vi "nanocal -- nuclear schottky goodness V5.vi"(5 "action":T1=enum."onlygrads", 6 "parameters IN":map{T2, dbl}(c390), 7 "weighting strategy":T3, 8 "dz/dω IN (V)":cdb[](array[numeric])=[1.7183506006211996e-05+0.0i, 1.7124360968751133e-05+0.0i, 1.7049104347380084e-05+0.0i, 1.700437896335042e-05+0.0i, 1.6984579723285106e-05+0.0i, 1.702277369054923e-05+0.0i, 1.713094025845651e-05+0.0i, 1.734249707866828e-05+0.0i, 1.768320429215342e-05+0.0i, 1.8195281152538477e-05+0.0i, 1.8917228661806973e-05+0.0i, 1.9897834564883332e-05+0.0i, 2.154104046962704e-05+0.0i, 2.3247799321765792e-05+0.0i, 2.5364678450551808e-05+0.0i, 2.8645788781885885e-05+0.0i, 3.204749554800641e-05+0.0i, 3.783559691555022e-05+0.0i, 4.245015867332296e-05+0.0i, 4.909131821431355e-05+0.0i, 5.511821898441184e-05+0.0i, 6.178843506022867e-05+0.0i, 7.1079604965352e-05+0.0i, 7.922304381453334e-05+0.0i, 8.814778883893872e-05+0.0i, 9.806709148886077e-05+0.0i, 0.00011119043245647465+0.0i, 0.00012253184919712196+0.0i, 0.00013777724317049346+0.0i, 0.0001508081004573332+0.0i, 0.00016547294918783876+0.0i, 0.00018003847596605868+0.0i, 0.00019518361086534857+0.0i, 0.00021134179818259658+0.0i, 0.0002372041782935464+0.0i, 0.00025518143132024254+0.0i, 0.0002835129702467886+0.0i, 0.0003060118087631287+0.0i, 0.00032860772064336976+0.0i, 0.0003492674091322389+0.0i, 0.00037498324855458583+0.0i, 0.00040021078021115026+0.0i, 0.00041969942568205823+0.0i, 0.00044367338947118773+0.0i, 0.0004634793607238068+0.0i, 0.00047921028781215815+0.0i, 0.0004880906353641744+0.0i, 0.0004932212623741357+0.0i, 0.000491476456593048+0.0i, 0.000480893803992059+0.0i, 0.0004535995818650303+0.0i, 0.000417087772881063+0.0i, 0.0003564148692854789+0.0i, 0.0003049201646356487+0.0i, 0.00021260191240459413+0.0i, 0.00011714858948470126+0.0i, 1.675457544365132e-05+0.0i, -6.8674075405897e-05+0.0i, -0.000156473047607305+0.0i, -0.00026709373934749337+0.0i, -0.0003544271565676041+0.0i, -0.00047937600197311275+0.0i, -0.0006086290582260493+0.0i, -0.0007031877411848573+0.0i, -0.0007564526901441745+0.0i, -0.000802489180995596+0.0i, -0.0008414596018105983+0.0i, -0.0008809346482248761+0.0i, -0.0009073902840241921+0.0i, -0.0009264953054508651+0.0i, -0.0009405659412141811+0.0i, -0.000951649722530156+0.0i, -0.0009557485581057351+0.0i, -0.0009558464741053665+0.0i, -0.0009509110176922098+0.0i, -0.0009411315169847015+0.0i, -0.0009303400913929496+0.0i, -0.0009171113529290538+0.0i, -0.0009022111527275027+0.0i, -0.0008813746494947608+0.0i, -0.0008581837971946129+0.0i, -0.0008372063466683705+0.0i, -0.0008165626610594428+0.0i, -0.0007901155435838691+0.0i, -0.0007682834352800848+0.0i, -0.000746231015527196+0.0i, -0.0007238798463130141+0.0i, -0.0007015567569177018+0.0i, -0.000679301954671598+0.0i, -0.0006572001413831251+0.0i, -0.000629855254567978+0.0i, -0.0006083942229188815+0.0i, -0.0005768631156754208+0.0i, -0.0005562177438951648+0.0i, -0.0005359092039599222+0.0i, -0.0005145186443378148+0.0i, -0.0004951602053444319+0.0i, -0.00047624970229075174+0.0i, -0.0004577401041527736+0.0i, -0.00043519037796120065+0.0i], 9 "Voltage IN (V)":cdb[](array[numeric])=[1.7183506006211996e-05+0.0i, 1.7124360968751133e-05+0.0i, 1.7049104347380084e-05+0.0i, 1.700437896335042e-05+0.0i, 1.6984579723285106e-05+0.0i, 1.702277369054923e-05+0.0i, 1.713094025845651e-05+0.0i, 1.734249707866828e-05+0.0i, 1.768320429215342e-05+0.0i, 1.8195281152538477e-05+0.0i, 1.8917228661806973e-05+0.0i, 1.9897834564883332e-05+0.0i, 2.154104046962704e-05+0.0i, 2.3247799321765792e-05+0.0i, 2.5364678450551808e-05+0.0i, 2.8645788781885885e-05+0.0i, 3.204749554800641e-05+0.0i, 3.783559691555022e-05+0.0i, 4.245015867332296e-05+0.0i, 4.909131821431355e-05+0.0i, 5.511821898441184e-05+0.0i, 6.178843506022867e-05+0.0i, 7.1079604965352e-05+0.0i, 7.922304381453334e-05+0.0i, 8.814778883893872e-05+0.0i, 9.806709148886077e-05+0.0i, 0.00011119043245647465+0.0i, 0.00012253184919712196+0.0i, 0.00013777724317049346+0.0i, 0.0001508081004573332+0.0i, 0.00016547294918783876+0.0i, 0.00018003847596605868+0.0i, 0.00019518361086534857+0.0i, 0.00021134179818259658+0.0i, 0.0002372041782935464+0.0i, 0.00025518143132024254+0.0i, 0.0002835129702467886+0.0i, 0.0003060118087631287+0.0i, 0.00032860772064336976+0.0i, 0.0003492674091322389+0.0i, 0.00037498324855458583+0.0i, 0.00040021078021115026+0.0i, 0.00041969942568205823+0.0i, 0.00044367338947118773+0.0i, 0.0004634793607238068+0.0i, 0.00047921028781215815+0.0i, 0.0004880906353641744+0.0i, 0.0004932212623741357+0.0i, 0.000491476456593048+0.0i, 0.000480893803992059+0.0i, 0.0004535995818650303+0.0i, 0.000417087772881063+0.0i, 0.0003564148692854789+0.0i, 0.0003049201646356487+0.0i, 0.00021260191240459413+0.0i, 0.00011714858948470126+0.0i, 1.675457544365132e-05+0.0i, -6.8674075405897e-05+0.0i, -0.000156473047607305+0.0i, -0.00026709373934749337+0.0i, -0.0003544271565676041+0.0i, -0.00047937600197311275+0.0i, -0.0006086290582260493+0.0i, -0.0007031877411848573+0.0i, -0.0007564526901441745+0.0i, -0.000802489180995596+0.0i, -0.0008414596018105983+0.0i, -0.0008809346482248761+0.0i, -0.0009073902840241921+0.0i, -0.0009264953054508651+0.0i, -0.0009405659412141811+0.0i, -0.000951649722530156+0.0i, -0.0009557485581057351+0.0i, -0.0009558464741053665+0.0i, -0.0009509110176922098+0.0i, -0.0009411315169847015+0.0i, -0.0009303400913929496+0.0i, -0.0009171113529290538+0.0i, -0.0009022111527275027+0.0i, -0.0008813746494947608+0.0i, -0.0008581837971946129+0.0i, -0.0008372063466683705+0.0i, -0.0008165626610594428+0.0i, -0.0007901155435838691+0.0i, -0.0007682834352800848+0.0i, -0.000746231015527196+0.0i, -0.0007238798463130141+0.0i, -0.0007015567569177018+0.0i, -0.000679301954671598+0.0i, -0.0006572001413831251+0.0i, -0.000629855254567978+0.0i, -0.0006083942229188815+0.0i, -0.0005768631156754208+0.0i, -0.0005562177438951648+0.0i, -0.0005359092039599222+0.0i, -0.0005145186443378148+0.0i, -0.0004951602053444319+0.0i, -0.00047624970229075174+0.0i, -0.0004577401041527736+0.0i, -0.00043519037796120065+0.0i], 10 "ω (rad/sec)":dbl[](array[numeric])=[32012.991918577427, 32390.261658505893, 32466.39798177853, 32499.14340521798, 32517.39286113775, 32529.046092051318, 32537.14525712326, 32543.111142615544, 32547.696343954158, 32551.33675949651, 32554.302325209504, 32556.769142360055, 32558.856995237307, 32560.650202739795, 32562.209843476354, 32563.58125099723, 32564.7987833122, 32565.88895894197, 32566.872575330308, 32567.766175404246, 32568.583086316496, 32569.334166794306, 32570.02835688638, 32570.673085530187, 32571.274580490695, 32571.838104118455, 32572.36813539066, 32572.868514009202, 32573.342552524307, 32573.793126289274, 32574.222746575288, 32574.633618125405, 32575.027687968828, 32575.40668442971, 32575.772149741057, 32576.12546690325, 32576.467883345118, 32576.800529469096, 32577.124435064776, 32577.440543590797, 32577.749724325146, 32578.052781957467, 32578.35046682089, 32578.643482565894, 32578.932492128843, 32579.218126471686, 32579.500987779396, 32579.781656707495, 32580.06069600583, 32580.338656060805, 32580.616078519142, 32580.89350097748, 32581.171461032456, 32581.45050033079, 32581.73116925889, 32582.0140305666, 32582.29966469628, 32582.58867447239, 32582.88169000423, 32583.179375080817, 32583.48243271314, 32583.791613234323, 32584.10772197351, 32584.43162756919, 32584.764273480003, 32585.106690135035, 32585.460007297228, 32585.825472395412, 32586.204468856296, 32586.59853891288, 32587.009410462997, 32587.439030535847, 32587.889604513977, 32588.363642815923, 32588.86402143446, 32589.39405291983, 32589.957576334426, 32590.559071508098, 32591.203800151903, 32591.897990030815, 32592.64907072179, 32593.46598163404, 32594.359581707977, 32595.343197883154, 32596.433373726086, 32597.650906041054, 32599.022313348767, 32600.58195429849, 32602.375161800977, 32604.46301467823, 32606.929831615616, 32609.895397541775, 32613.535812870963, 32618.12101442274, 32624.086899701866, 32632.186064986967, 32643.839295900536, 32662.088751820305, 32694.834175046595, 32770.97049853239]) -> (0 "R norm":dbl=-1.0, 1 "G":dbl=-1.0, 2 "R(ω) out":cdb[](array[numeric])=[1.7183506006211996e-05+0.0i, 1.7124360968751133e-05+0.0i, 1.7049104347380084e-05+0.0i, 1.700437896335042e-05+0.0i, 1.6984579723285106e-05+0.0i, 1.702277369054923e-05+0.0i, 1.713094025845651e-05+0.0i, 1.734249707866828e-05+0.0i, 1.768320429215342e-05+0.0i, 1.8195281152538477e-05+0.0i, 1.8917228661806973e-05+0.0i, 1.9897834564883332e-05+0.0i, 2.154104046962704e-05+0.0i, 2.3247799321765792e-05+0.0i, 2.5364678450551808e-05+0.0i, 2.8645788781885885e-05+0.0i, 3.204749554800641e-05+0.0i, 3.783559691555022e-05+0.0i, 4.245015867332296e-05+0.0i, 4.909131821431355e-05+0.0i, 5.511821898441184e-05+0.0i, 6.178843506022867e-05+0.0i, 7.1079604965352e-05+0.0i, 7.922304381453334e-05+0.0i, 8.814778883893872e-05+0.0i, 9.806709148886077e-05+0.0i, 0.00011119043245647465+0.0i, 0.00012253184919712196+0.0i, 0.00013777724317049346+0.0i, 0.0001508081004573332+0.0i, 0.00016547294918783876+0.0i, 0.00018003847596605868+0.0i, 0.00019518361086534857+0.0i, 0.00021134179818259658+0.0i, 0.0002372041782935464+0.0i, 0.00025518143132024254+0.0i, 0.0002835129702467886+0.0i, 0.0003060118087631287+0.0i, 0.00032860772064336976+0.0i, 0.0003492674091322389+0.0i, 0.00037498324855458583+0.0i, 0.00040021078021115026+0.0i, 0.00041969942568205823+0.0i, 0.00044367338947118773+0.0i, 0.0004634793607238068+0.0i, 0.00047921028781215815+0.0i, 0.0004880906353641744+0.0i, 0.0004932212623741357+0.0i, 0.000491476456593048+0.0i, 0.000480893803992059+0.0i, 0.0004535995818650303+0.0i, 0.000417087772881063+0.0i, 0.0003564148692854789+0.0i, 0.0003049201646356487+0.0i, 0.00021260191240459413+0.0i, 0.00011714858948470126+0.0i, 1.675457544365132e-05+0.0i, -6.8674075405897e-05+0.0i, -0.000156473047607305+0.0i, -0.00026709373934749337+0.0i, -0.0003544271565676041+0.0i, -0.00047937600197311275+0.0i, -0.0006086290582260493+0.0i, -0.0007031877411848573+0.0i, -0.0007564526901441745+0.0i, -0.000802489180995596+0.0i, -0.0008414596018105983+0.0i, -0.0008809346482248761+0.0i, -0.0009073902840241921+0.0i, -0.0009264953054508651+0.0i, -0.0009405659412141811+0.0i, -0.000951649722530156+0.0i, -0.0009557485581057351+0.0i, -0.0009558464741053665+0.0i, -0.0009509110176922098+0.0i, -0.0009411315169847015+0.0i, -0.0009303400913929496+0.0i, -0.0009171113529290538+0.0i, -0.0009022111527275027+0.0i, -0.0008813746494947608+0.0i, -0.0008581837971946129+0.0i, -0.0008372063466683705+0.0i, -0.0008165626610594428+0.0i, -0.0007901155435838691+0.0i, -0.0007682834352800848+0.0i, -0.000746231015527196+0.0i, -0.0007238798463130141+0.0i, -0.0007015567569177018+0.0i, -0.000679301954671598+0.0i, -0.0006572001413831251+0.0i, -0.000629855254567978+0.0i, -0.0006083942229188815+0.0i, -0.0005768631156754208+0.0i, -0.0005562177438951648+0.0i, -0.0005359092039599222+0.0i, -0.0005145186443378148+0.0i, -0.0004951602053444319+0.0i, -0.00047624970229075174+0.0i, -0.0004577401041527736+0.0i, -0.00043519037796120065+0.0i], 3 "dG / d log α   OUT":map{T2, dbl}(c390))   [LabVIEW 2021]
uses:
  nanocal-goodness-weighting-strategy.ctl
  3-lorentzian-parameters.ctl
  3-lorentzian-heat-response action.ctl
  <vilib>/Utility/miscctls.llb/LVMapReplaceAction.ctl
  <vilib>/Analysis/_algsub.llb/Matrix Norm Type.ctl
  <vilib>/Analysis/baseanly.llb/Matrix Type of Inverse Matrix.ctl
  <vilib>/Analysis/baseanly.llb/Real A x B.vi
  <vilib>/Analysis/_algsub.llb/Real Matrix Norm.vi
  <vilib>/Analysis/Matrix/Numeric/Conversions/Array To Matrix - RA2.vi
  <vilib>/Analysis/baseanly.llb/Real Inverse Matrix.vi
  <vilib>/Analysis/Matrix/Numeric/Conversions/Array To Matrix - RA.vi
  <vilib>/Analysis/Matrix/Numeric/Conversions/Matrix To Array - RM.vi
  <vilib>/Analysis/Matrix/NI_Matrix.lvlib
  <vilib>/Analysis/NI_AALBase.lvlib
  <vilib>/Analysis/NI_AALPro.lvlib
panel:
  out "d2G / d log α d log  β  matrix OUT":dbl[](array[numeric])
  out "d2G / d log α d log  β  map  OUT":map{i32[], dbl}(c390)
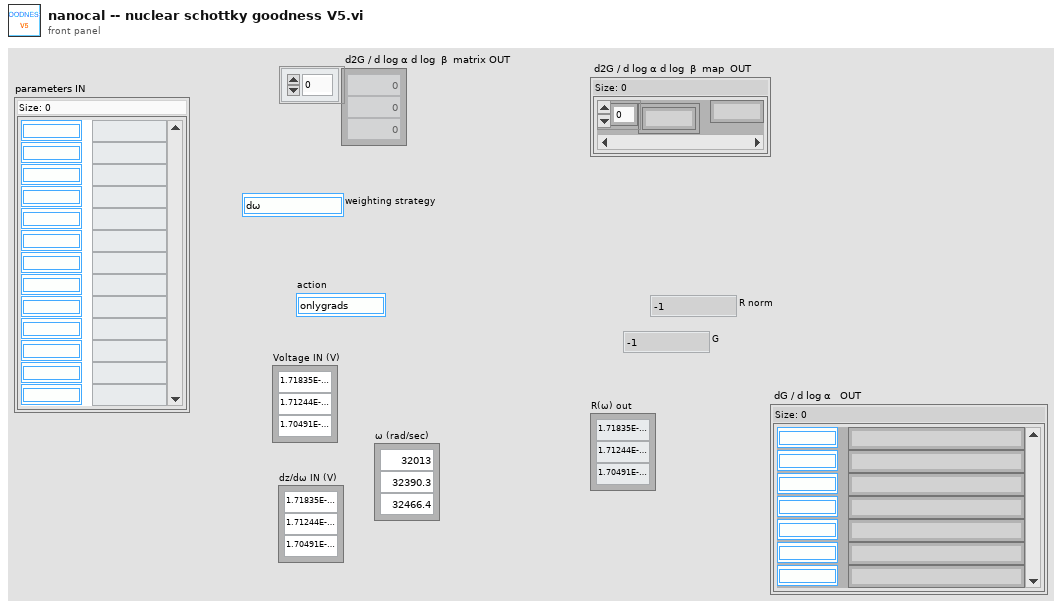
[diagram p1: front panel]
types:
  T1 = typedef "3-lorentzian-heat-response action.ctl" = enum16{"calc R", "create string", "calc m1m2m3", "dζ", "dT1", "dτS", "dτN", "dτC", "d-all", "dκ0", "T(K)", "m1", "m2", "m3", "parse string", "θ (deg)", "B (T)", "onlygrads", "newton", "create emty string"}
  T2 = typedef "3-lorentzian-parameters.ctl" = enum16{"ζ", "τ1", "τS", "τN", "τC", "κ0", "m1", "m2", "m3", "T (K)", "B (T)", "θ (deg)", "side (S|R)", "set of (B|T)", "Re(offset)", "Im(offset)", "στ1", "στ1-", "στ1+", "στS", "στS-", "στS+", "στN", "στN-", "στN+"}
  T3 = typedef "nanocal-goodness-weighting-strategy.ctl" = enum16{"dω", "dω √(|dz/dω|)", "dω |dz/dω|", "phase", "andreas", "sum", "1/f noise"}
  T4 = typedef "LVMapReplaceAction.ctl" = enum32{"Modify Entry only if found", "Add or Modify Entry", "Delete Entry"}
  T5 = typedef "NI_AALBase.lvlib/Matrix Type of Inverse Matrix.ctl" = enum32{"General", "Positive Definite", "Lower Triangular", "Upper Triangular"}
  T6 = typedef "NI_AALPro.lvlib/Matrix Norm Type.ctl" = i32
  T7 = typedef "NI_Matrix.lvlib/RealMatrix.ctl" = dbl[][]
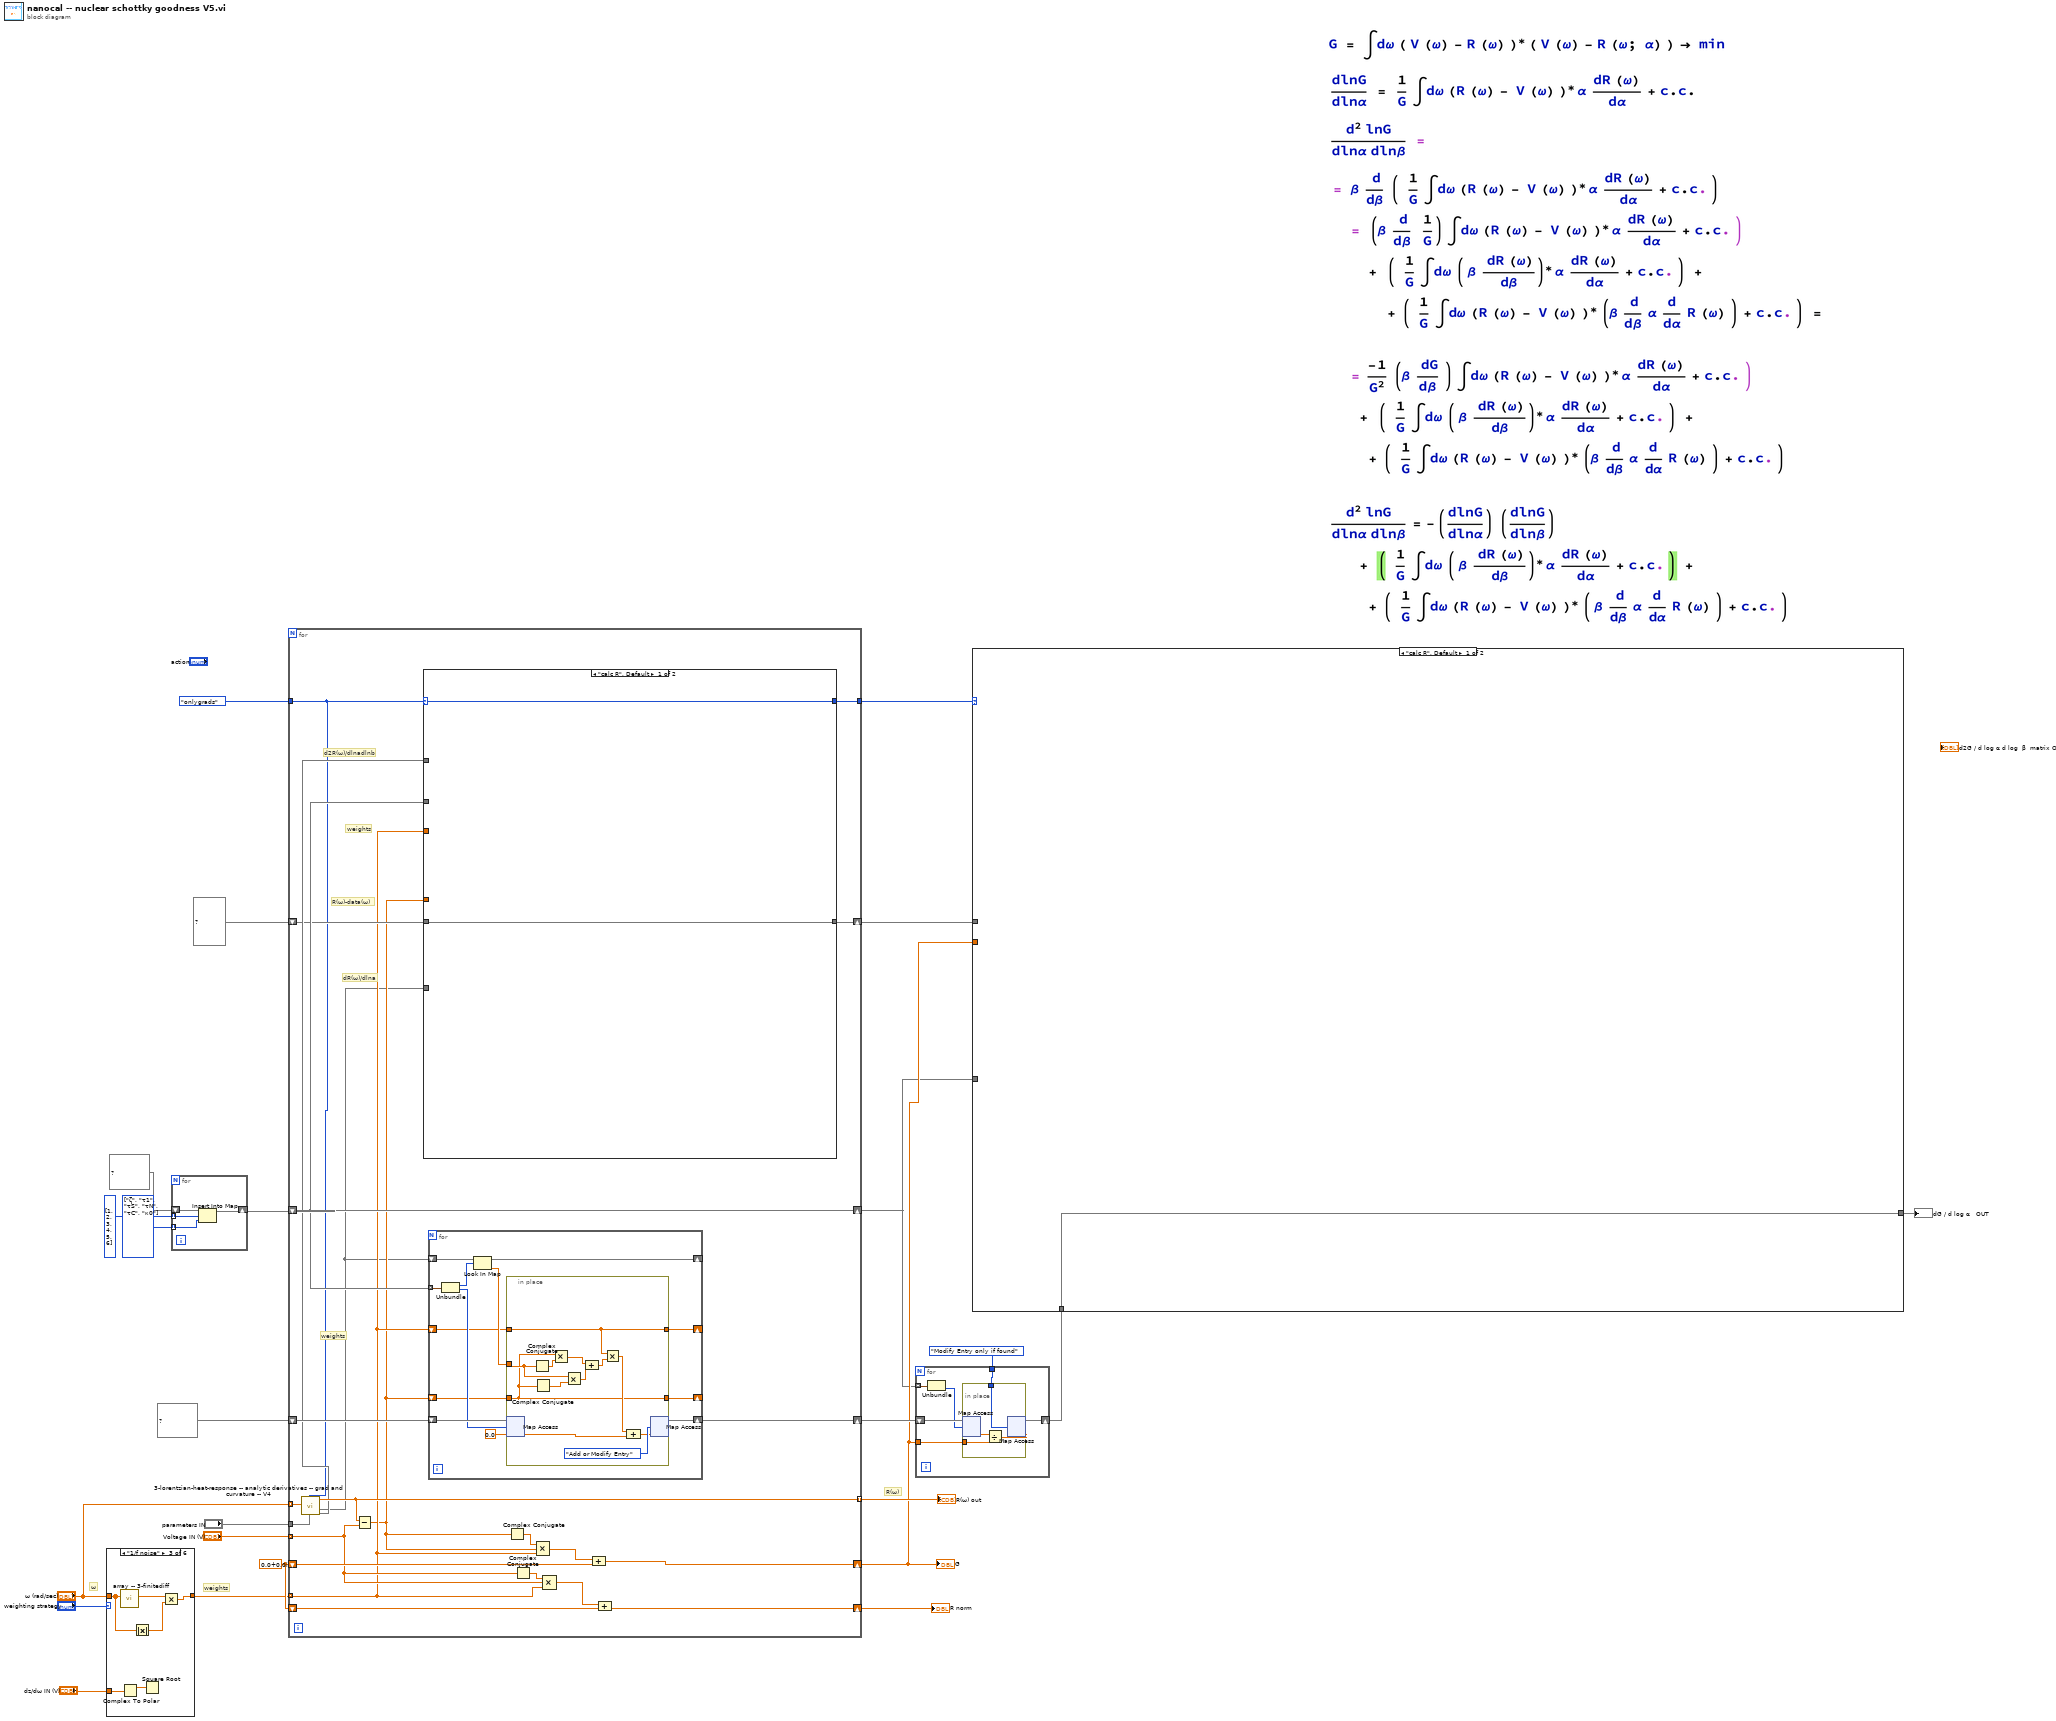
[diagram p0: block diagram]
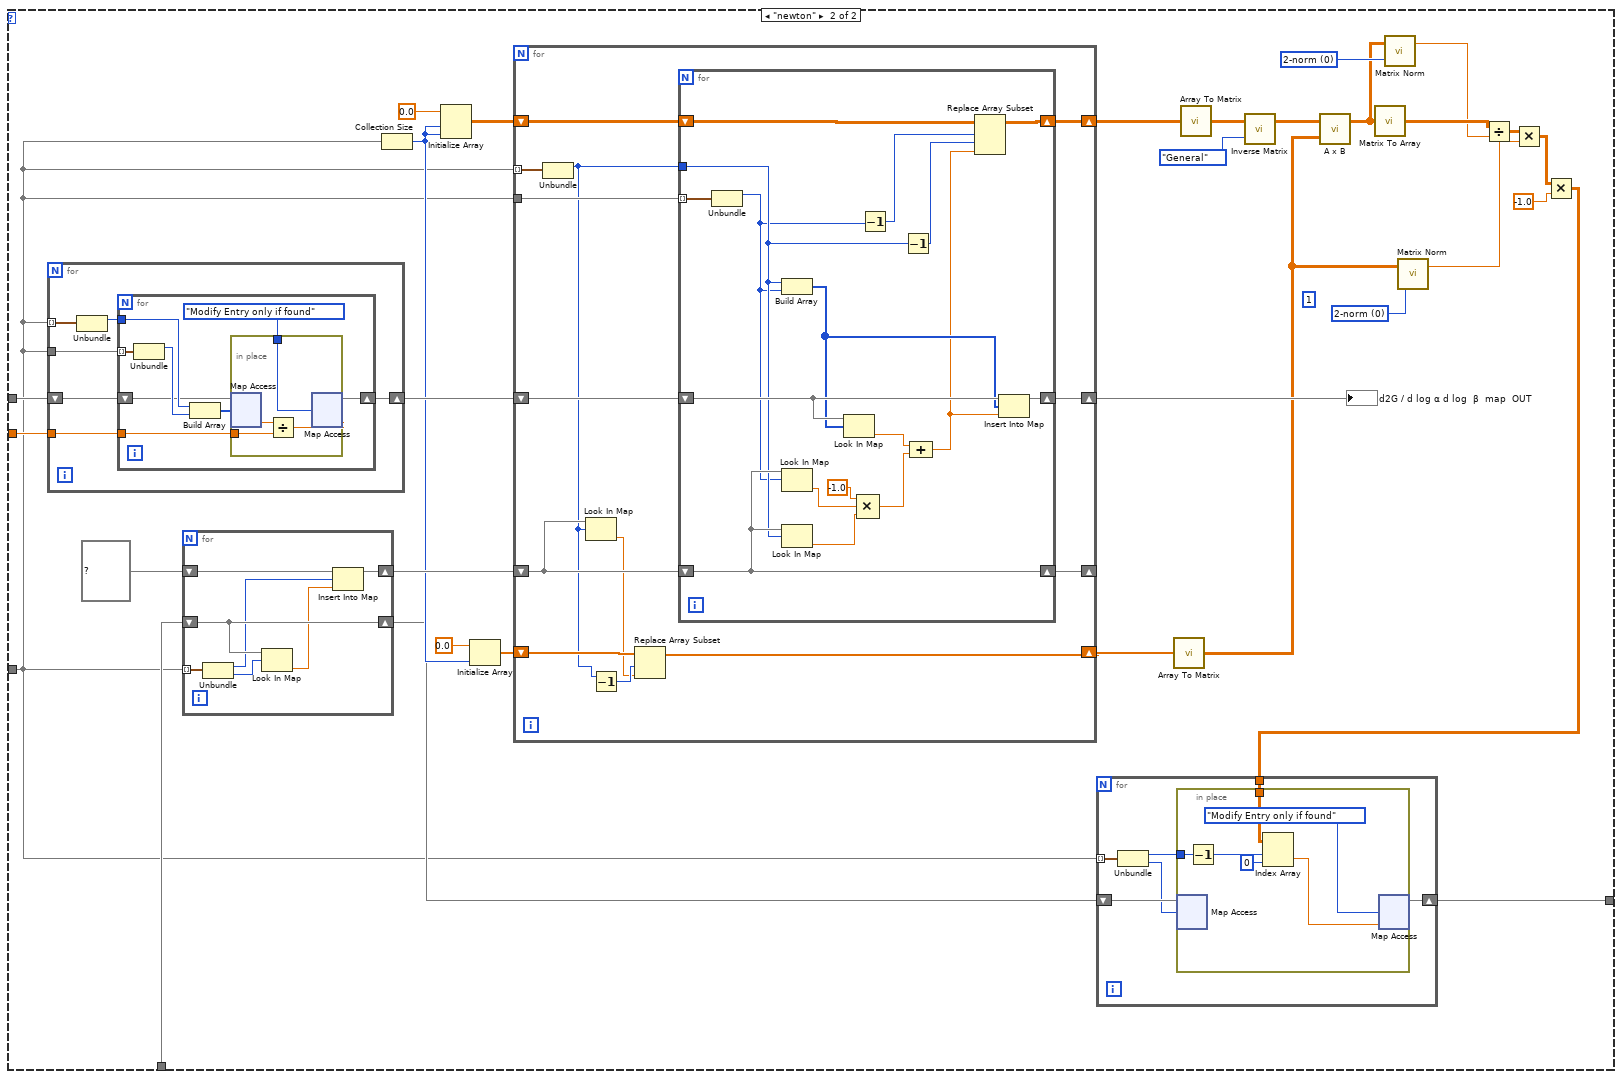
[diagram p2: hidden frame]
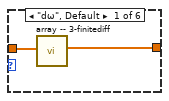
[diagram p3: hidden frame]
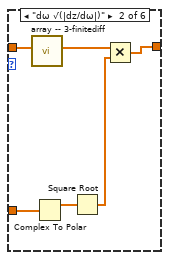
[diagram p4: hidden frame]
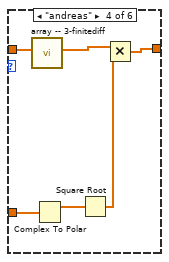
[diagram p5: hidden frame]
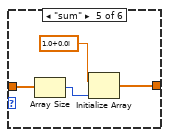
[diagram p6: hidden frame]
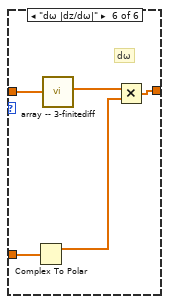
[diagram p7: hidden frame]
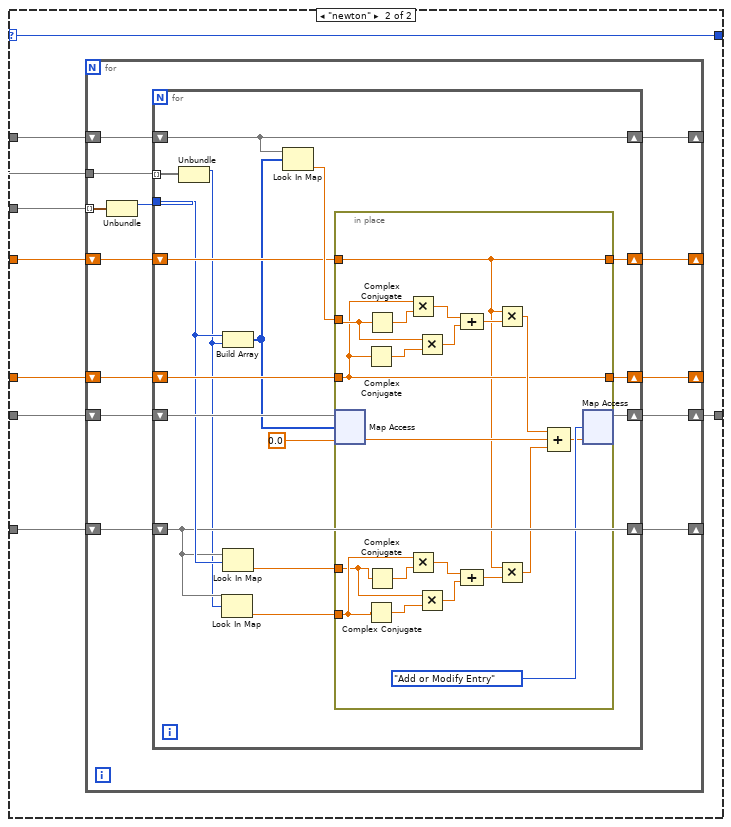
[diagram p8: hidden frame]
diagram:
  w14 = cdb 0.0+0.0i ("y")
  w19 = T2[] [enum."ζ", enum."τ1", enum."τS", enum."τN", enum."τC", enum."κ0"] items=["ζ", "τ1", "τS", "τN", "τC", "κ0", "m1", "m2", "m3", "T (K)", "B (T)", "θ (deg)", "side (S|R)", "set of (B|T)", "Re(offset)", "Im(offset)", "στ1", "στ1-", "στ1+", "στS", "στS-", "στS+", "στN", "στN-", "στN+"]
  # "weights"
  # "R(ω)"
  # "ω"
  n1 = case shown="\"1/f noise\"" "weighting strategy" {
    tunnel: "dz/dω IN (V)" -> [_ w32 w38 w44 _ w53]
    tunnel: "ω (rad/sec)" -> [w26 w28 w34 w40 w48 w52]
    tunnel: [w25 w27 w35 w39 w45 w49] -> w2
    frame "dω", Default {
      n2 = call "array -- 3-finitediff.vi"("ω (rad/sec)"=w26) -> ("dω (rad/sec)"=w25:cdb[])  [unwired: 10 in]
    }
    frame "dω √(|dz/dω|)" {
      n3 = call "array -- 3-finitediff.vi"("ω (rad/sec)"=w28) -> ("dω (rad/sec)"=w30:cdb[])  [unwired: 10 in]
      n4 = Complex To Polar(r * e^(i*theta)=w32) -> (r=w31:dbl[])  [unwired: 1 out]
      n5 = Square Root(x=w31) -> (sqrt(x)=w29:dbl[])
      n6 = Multiply(x=w30, y=w29) -> (x*y=w27:cdb[])
    }
    frame "1/f noise" {
      n7 = call "array -- 3-finitediff.vi"("ω (rad/sec)"=w34) -> ("dω (rad/sec)"=w36:cdb[])  [unwired: 10 in]
      n8 = Complex To Polar(r * e^(i*theta)=w38) -> (r=w37:dbl[])  [unwired: 1 out]
      n9 = Absolute Value(x=w34) -> (abs(x)=w33:dbl[])
      n10 = Square Root(x=w37) -> ()  [unwired: 1 out]
      n11 = Multiply(x=w36, y=w33) -> (x*y=w35:cdb[])
    }
    frame "andreas" {
      n12 = call "array -- 3-finitediff.vi"("ω (rad/sec)"=w40) -> ("dω (rad/sec)"=w42:cdb[])  [unwired: 10 in]
      n13 = Complex To Polar(r * e^(i*theta)=w44) -> (r=w43:dbl[])  [unwired: 1 out]
      n14 = Square Root(x=w43) -> (sqrt(x)=w41:dbl[])
      n15 = Multiply(x=w42, y=w41) -> (x*y=w39:cdb[])
    }
    frame "sum" {
      n16 = Array Size(array=w48) -> (size(s)=w47:i32)
      n17 = Initialize Array(cdb 1.0+0.0i ("y"), w47) -> (w45:cdb[])
    }
    frame "dω |dz/dω|" {
      # "dω"
      n18 = Complex To Polar(r * e^(i*theta)=w53) -> (r=w51:dbl[])  [unwired: 1 out]
      n19 = call "array -- 3-finitediff.vi"("ω (rad/sec)"=w52) -> ("dω (rad/sec)"=w50:cdb[])  [unwired: 10 in]
      n20 = Multiply(x=w50, y=w51) -> (x*y=w49:cdb[])
    }
  }
  n21 = for {
    tunnel: w19 -> [w54] mode=indexing
    shift-right: [w56] -> w12
    shift-left: map{i32, T2} {} ("parameters IN") -> [w57]
    tunnel: i32[] [1, 2, 3, 4, 5, 6] -> [w55] mode=indexing
    n22 = Insert Into Map(map in=w57, key=w55, value=w54) -> (map out=w56:map{i32, T2})  [unwired: 2 out]
  }
  n23 = for {
    tunnel: "ω (rad/sec)" -> [w79] mode=indexing
    tunnel: [w78] -> w21 mode=indexing
    tunnel: "parameters IN" -> [w80]
    tunnel: "Voltage IN (V)" -> [w67] mode=indexing
    tunnel: w2 -> [w62] mode=indexing
    shift-right: [w76] -> w15
    shift-left: map{T2, dbl} {} ("parameters IN") -> [w77]
    shift-right: [w66] -> w7
    shift-left: w12 -> [w66]
    shift-right: [w72] -> w8
    shift-left: w14 -> [w73]
    shift-right: [w68] -> w13
    shift-left: w14 -> [w69]
    shift-right: [w63] -> w9
    shift-left: map{i32[], dbl} {} ("parameters IN") -> [w64]
    tunnel: 3-lorentzian-heat-response_action."onlygrads" ("action") -> [w59]
    tunnel: [w58] -> w4
    # "R(ω)-data(ω)"
    # "weights"
    # "dR(ω)/dlna"
    # "d2R(ω)/dlnadlnb"
    # "weights"
    n24 = call "3-lorentzian-heat-response -- analytic derivatives -- grad and curvature -- V4.vi"("parameters map  IN"=w80, "action"=w59, "ω (rad/sec)"=w79) -> ("second derivatives map out"=w65:map{i32[], cdb}, "grad map  out"=w60:map{i32, cdb}, "R(ω)"=w78:cdb)  [unwired: 5 in, 1 out]
    n25 = Subtract(x=w78, y=w67) -> (x-y=w61:cdb)
    n26 = case shown="\"calc R\", Default" w59 {
      selector: w59 -> [w81 w83]
      tunnel: w66 -> [_ w90]
      tunnel: w65 -> [_ w89]
      tunnel: w64 -> [w82 w88]
      tunnel: [w82 w87] -> w63
      tunnel: w62 -> [_ w86]
      tunnel: w61 -> [_ w85]
      tunnel: w60 -> [_ w84]
      tunnel: [w81 w83] -> w58
      frame "calc R", Default {
      }
      frame "newton" {
        n27 = for {
          shift-right: [w103] -> w87
          shift-left: w88 -> [w102]
          shift-right: [w101] -> _
          shift-left: w86 -> [w99]
          shift-right: [w100] -> _
          shift-left: w85 -> [w98]
          shift-right: [w97] -> _
          shift-left: w89 -> [w96]
          tunnel: w90 -> [w95] mode=indexing
          tunnel: w90 -> [w94]
          shift-right: [w91] -> _
          shift-left: w84 -> [w92]
          n28 = Unbundle(w95) -> ("index"=w93:i32)  [unwired: 1 out]
          n29 = for {
            shift-right: [w119] -> w97
            shift-left: w96 -> [w119]
            shift-right: [w116] -> w100
            shift-left: w98 -> [w115]
            shift-right: [w113] -> w103
            shift-left: w102 -> [w118]
            tunnel: w94 -> [w110] mode=indexing
            shift-right: [w111] -> w101
            shift-left: w99 -> [w112]
            tunnel: w93 -> [w108]
            shift-right: [w107] -> w91
            shift-left: w92 -> [w107]
            n30 = Unbundle(w110) -> ("index"=w106:i32)  [unwired: 1 out]
            n31 = Look In Map(map=w107, key=w106) -> (value=w104:cdb)  [unwired: 1 in, 1 out]
            n32 = Build Array(w108, w106) -> (w109:i32[])
            n33 = Look In Map(map=w107, key=w108) -> (value=w105:cdb)  [unwired: 1 in, 1 out]
            n34 = Look In Map(map=w119, key=w109) -> (value=w114:cdb)  [unwired: 1 in, 1 out]
            n35 = in-place {
              in-place-border: [w129] -> w116
              in-place-border: w115 -> [w129]
              in-place-border: w114 -> [w136]
              in-place-border: w112 -> [w121]
              in-place-border: [w121] -> w111
              in-place-border: w105 -> [w122]
              in-place-border: w104 -> [w123]
              n36 = in-place-map #1(w118, w109, 0.0 ("number")) -> (w135:dbl)  [unwired: 1 out]
              n37 = Complex Conjugate(1:w129) -> (0:w137:cdb)
              n38 = Complex Conjugate(1:w123) -> (0:w127:cdb)
              n39 = Complex Conjugate(1:w136) -> (0:w138:cdb)
              n40 = Complex Conjugate(1:w122) -> (0:w128:cdb)
              n41 = Multiply(x=w129, y=w138) -> (x*y=w133:cdb)
              n42 = Multiply(x=w123, y=w128) -> (x*y=w126:cdb)
              n43 = Multiply(x=w136, y=w137) -> (x*y=w132:cdb)
              n44 = Multiply(x=w122, y=w127) -> (x*y=w125:cdb)
              n45 = Compound Arithmetic op=ADD(w133, w132) -> (w131:cdb)
              n46 = Compound Arithmetic op=ADD(w126, w125) -> (w124:cdb)
              n47 = Multiply(x=w121, y=w131) -> (x*y=w130:cdb)
              n48 = Multiply(x=w121, y=w124) -> (x*y=w120:cdb)
              n49 = Compound Arithmetic op=ADD(w130, w135, w120) -> (w134:cdb)
              n50 = in-place-map #1(w134, LVMapReplaceAction."Add or Modify Entry" ("action")) -> (w113:map{i32[], dbl})  [unwired: 2 out]
            }
          }
        }
      }
    }
    n51 = for {
      shift-right: [w151] -> _
      shift-left: w60 -> [w151]
      shift-right: [w145] -> _
      shift-left: w61 -> [w144]
      shift-right: [w142] -> w76
      shift-left: w77 -> [w148]
      tunnel: w66 -> [w150] mode=indexing
      shift-right: [w140] -> _
      shift-left: w62 -> [w141]
      n52 = Unbundle(w150) -> ("index"=w149:i32, "X selector"=w147:T2)
      n53 = Look In Map(map=w151, key=w149) -> (value=w143:cdb)  [unwired: 1 in, 1 out]
      n54 = in-place {
        in-place-border: [w153] -> w145
        in-place-border: w144 -> [w153]
        in-place-border: w143 -> [w160]
        in-place-border: w141 -> [w152]
        in-place-border: [w152] -> w140
        n55 = in-place-map #2(w148, w147, 0.0 ("number")) -> (w159:dbl)  [unwired: 1 out]
        n56 = Complex Conjugate(1:w160) -> (0:w162:cdb)
        n57 = Complex Conjugate(1:w153) -> (0:w161:cdb)
        n58 = Multiply(x=w153, y=w162) -> (x*y=w157:cdb)
        n59 = Multiply(x=w160, y=w161) -> (x*y=w156:cdb)
        n60 = Compound Arithmetic op=ADD(w157, w156) -> (w155:cdb)
        n61 = Multiply(x=w152, y=w155) -> (x*y=w154:cdb)
        n62 = Compound Arithmetic op=ADD(w154, w159) -> (w158:cdb)
        n63 = in-place-map #2(w158, LVMapReplaceAction."Add or Modify Entry" ("action")) -> (w142:map{T2, dbl})  [unwired: 2 out]
      }
    }
    n64 = Complex Conjugate(1:w61) -> (0:w75:cdb)
    n65 = Complex Conjugate(1:w67) -> (0:w71:cdb)
    n66 = Compound Arithmetic op=MULTIPLY(w75, w61, w62) -> (w74:cdb)
    n67 = Compound Arithmetic op=MULTIPLY(w71, w67, w62) -> (w70:cdb)
    n68 = Compound Arithmetic op=ADD(w74, w73) -> (w72:cdb)
    n69 = Compound Arithmetic op=ADD(w70, w69) -> (w68:cdb)
  }
  "G" <- w8
  "R norm" <- w13
  "R(ω) out" <- w21
  n70 = for {
    tunnel: w7 -> [w166] mode=indexing
    shift-right: [w168] -> w10
    shift-left: w15 -> [w169]
    tunnel: w8 -> [w167]
    tunnel: LVMapReplaceAction."Modify Entry only if found" ("action") -> [w164]
    n71 = Unbundle(w166) -> ("X selector"=w165:T2)  [unwired: 1 out]
    n72 = in-place {
      in-place-border: w167 -> [w172]
      in-place-border: w164 -> [w170]
      n73 = in-place-map #3(w169, w165) -> (w173:dbl)  [unwired: 1 in, 1 out]
      n74 = Divide(x=w173, y=w172) -> (x/y=w171:cdb)
      n75 = in-place-map #3(w171, w170) -> (w168:map{T2, dbl})  [unwired: 2 out]
    }
  }
  n76 = case shown="\"calc R\", Default" w4 {
    tunnel: w10 -> [w174 w204]
    tunnel: w9 -> [_ w203]
    tunnel: w8 -> [_ w201]
    tunnel: w7 -> [_ w183]
    tunnel: [w174 w182] -> w6
    frame "calc R", Default {
    }
    frame "newton" {
      w189 = T6 0 items=["2-norm", "1-norm", "F-norm", "Inf-norm"] ("norm type")
      w190 = T6 0 items=["2-norm", "1-norm", "F-norm", "Inf-norm"] ("norm type")
      (unwired) 1 ("number of columns")
      n77 = for {
        tunnel: w183 -> [w222] mode=indexing
        tunnel: w183 -> [w223]
        shift-right: [w219] -> w202
        shift-left: w203 -> [w220]
        tunnel: w201 -> [w218]
        n78 = Unbundle(w222) -> ("index"=w221:i32)  [unwired: 1 out]
        n79 = for {
          tunnel: w223 -> [w231] mode=indexing
          tunnel: w221 -> [w230]
          shift-right: [w227] -> w219
          shift-left: w220 -> [w228]
          tunnel: w218 -> [w225]
          n80 = Unbundle(w231) -> ("index"=w229:i32)  [unwired: 1 out]
          n81 = Build Array(w230, w229) -> (w226:i32[])
          n82 = in-place {
            in-place-border: w225 -> [w234]
            in-place-border: LVMapReplaceAction."Modify Entry only if found" ("action") -> [w232]
            n83 = in-place-map #4(w228, w226) -> (w235:dbl)  [unwired: 1 in, 1 out]
            n84 = Divide(x=w235, y=w234) -> (x/y=w233:cdb)
            n85 = in-place-map #4(w233, w232) -> (w227:map{i32[], dbl})  [unwired: 2 out]
          }
        }
      }
      n86 = for {
        shift-right: [w271] -> w200
        shift-left: map{i32, dbl} {} ("parameters IN") -> [w272]
        tunnel: w183 -> [w270] mode=indexing
        shift-right: [w269] -> w184
        shift-left: w204 -> [w269]
        n87 = Unbundle(w270) -> ("index"=w267:i32, "X selector"=w268:T2)
        n88 = Look In Map(map=w269, key=w268) -> (value=w266:dbl)  [unwired: 1 in, 1 out]
        n89 = Insert Into Map(map in=w272, key=w267, value=w266) -> (map out=w271:map{i32, dbl})  [unwired: 2 out]
      }
      n90 = Collection Size(1:w183) -> (0:w191:i32)
      n91 = Initialize Array(0.0 ("number"), w191, w191) -> (w195:dbl[][])
      n92 = Initialize Array(0.0 ("number"), w191) -> (w198:dbl[])
      n93 = for {
        tunnel: w183 -> [w247] mode=indexing
        tunnel: w183 -> [w248]
        shift-right: [w245] -> w192
        shift-left: w202 -> [w246]
        shift-right: [w244] -> _
        shift-left: w200 -> [w242]
        shift-right: [w238] -> w196
        shift-left: w198 -> [w243]
        shift-right: [w237] -> w194
        shift-left: w195 -> [w236]
        n94 = Unbundle(w247) -> ("index"=w241:i32)  [unwired: 1 out]
        n95 = Look In Map(map=w242, key=w241) -> (value=w239:dbl)  [unwired: 1 in, 1 out]
        n96 = Decrement(x=w241) -> (x-1=w240:i32)
        n97 = Replace Array Subset(array=w243, new element=w239, index=w240) -> (w238:dbl[])
        n98 = for {
          tunnel: w248 -> [w265] mode=indexing
          tunnel: w241 -> [w254]
          shift-right: [w257] -> w245
          shift-left: w246 -> [w258]
          shift-right: [w264] -> w244
          shift-left: w242 -> [w264]
          shift-right: [w255] -> w237
          shift-left: w236 -> [w249]
          n99 = Unbundle(w265) -> ("index"=w253:i32)  [unwired: 1 out]
          n100 = Build Array(w254, w253) -> (w256:i32[])
          n101 = Look In Map(map=w264, key=w253) -> (value=w262:dbl)  [unwired: 1 in, 1 out]
          n102 = Look In Map(map=w264, key=w254) -> (value=w263:dbl)  [unwired: 1 in, 1 out]
          n103 = Look In Map(map=w258, key=w256) -> (value=w260:dbl)  [unwired: 1 in, 1 out]
          n104 = Compound Arithmetic op=MULTIPLY(-1.0 ("value"), w262, w263) -> (w259:dbl)
          n105 = Decrement(x=w253) -> (x-1=w252:i32)
          n106 = Decrement(x=w254) -> (x-1=w251:i32)
          n107 = Compound Arithmetic op=ADD(w260, w259) -> (w250:dbl)
          n108 = Replace Array Subset(array=w249, new element=w250, index (row)=w252, index (col)=w251) -> (w255:dbl[][])
          n109 = Insert Into Map(map in=w258, key=w256, value=w250) -> (map out=w257:map{i32[], dbl})  [unwired: 2 out]
        }
      }
      "d2G / d log α d log  β  map  OUT" <- w192
      n110 = call-poly <vilib>:"Array To Matrix.vi"("Real 1D Array"=w196) -> ("Real Matrix (Column Vector)"=w175:T7)
      n111 = call-poly <vilib>:"Array To Matrix.vi"("Real 2D Array"=w194) -> ("Real Matrix"=w178:T7)
      n112 = call-poly <vilib>:"Inverse Matrix.vi"("matrix type"=Matrix_Type_of_Inverse_Matrix."General", "Input Matrix"=w178) -> ("Inverse Matrix"=w177:T7)  [unwired: 1 out]
      n113 = call-poly <vilib>:"A x B.vi"("B"=w175, "A"=w177) -> ("A x B"=w176:T7)  [unwired: 1 out]
      n114 = call-poly <vilib>:"Matrix To Array.vi"("Real Matrix"=w176) -> ("Real 2D Array"=w188:dbl[][])
      n115 = call-poly <vilib>:"Matrix Norm.vi"("norm type"=w190, "Input Matrix"=w176) -> ("norm"=w187:dbl)  [unwired: 1 out]
      n116 = call-poly <vilib>:"Matrix Norm.vi"("norm type"=w189, "Input Matrix"=w175) -> ("norm"=w185:dbl)  [unwired: 1 out]
      n117 = Divide(x=w188, y=w187) -> (x/y=w186:dbl[][])
      n118 = Multiply(x=w186, y=w185) -> (x*y=w181:dbl[][])
      n119 = Multiply(x=w181, y=-1.0) -> (x*y=w179:dbl[][])
      n120 = for {
        tunnel: w183 -> [w209] mode=indexing
        shift-right: [w210] -> w182
        shift-left: w184 -> [w211]
        tunnel: w179 -> [w207]
        n121 = Unbundle(w209) -> ("index"=w206:i32, "X selector"=w208:T2)
        n122 = in-place {
          in-place-border: w207 -> [w216]
          in-place-border: w206 -> [w215]
          n123 = in-place-map #5(w211, w208) -> ()  [unwired: 1 in, 2 out]
          n124 = Decrement(x=w215) -> (x-1=w214:i32)
          n125 = Index Array(array=w216, index (row)=w214, index (col)=0 ("disabled index (col)")) -> (element=w213:dbl)
          n126 = in-place-map #5(w213, LVMapReplaceAction."Modify Entry only if found" ("action")) -> (w210:map{T2, dbl})  [unwired: 2 out]
        }
      }
    }
  }
  "dG / d log α   OUT" <- w6
